vi "Fetch Background Measurements.vi"   [LabVIEW 2012, in "NH Research Regenerative Test Series.lvlib"]
doc: "Returns the most recent measurements that are always being made by the hardware in the background (except while a waveform capture is being made)."
uses:
  <instrlib>/NH Research Regenerative Test Series/NH Research Regenerative Test Series.lvlib
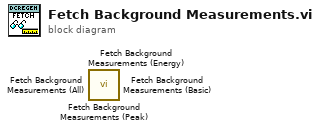
[diagram p0: block diagram]
diagram:
  n1 = call <instrlib>:"Fetch Background Measurements (Peak).vi"() -> ()  [unwired: 13 in, 3 out]
  n2 = call <instrlib>:"Fetch Background Measurements (Energy).vi"() -> ()  [unwired: 13 in, 3 out]
  n3 = call <instrlib>:"Fetch Background Measurements (All).vi"() -> ()  [unwired: 13 in, 3 out]
  n4 = call <instrlib>:"Fetch Background Measurements (Basic).vi"() -> ()  [unwired: 13 in, 3 out]
